vi "save digital settings.vi"(8 "error in (no error)":errorcluster, 11 "Digital Signal":T1={"DAQ Board Name"="DAQ_Simu1", "Port Digitales"=[], "rate"=1000.0, "Tiempo"=100}) -> (0 "error out":errorcluster)   [LabVIEW 2020, in "Settings.lvlib"]
uses:
  Settings.lvlib
  Digital typeSignal--cluster.ctl
  <vilib>/drjdpowell/SQLite Library/SQL Connection/Open (path).vi
  <vilib>/drjdpowell/SQLite Library/SQL Connection/Open (string).vi
  <vilib>/AdvancedString/Path To Command Line String.vi
  <vilib>/drjdpowell/SQLite Library/SQL Connection/Execute SQL (1D String).vi
  <vilib>/drjdpowell/SQLite Library/SQL Connection/Connection.lvclass
  <vilib>/drjdpowell/SQLite Library/SQLite.lvlib
panel:
  out "delimited string":string
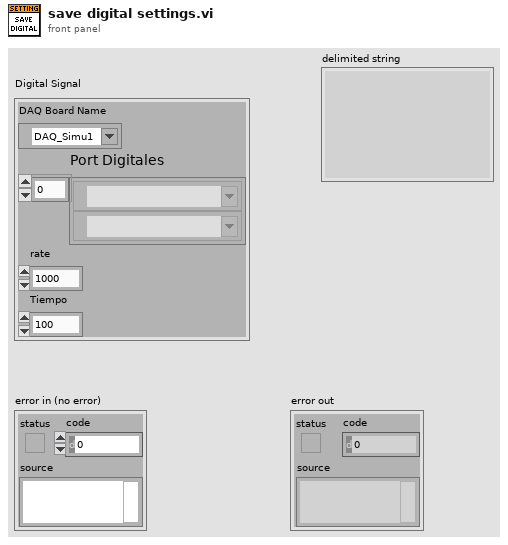
[diagram p1: front panel]
types:
  T1 = typedef "Digital typeSignal--cluster.ctl" = cluster{"DAQ Board Name":tag, "Port Digitales":tag[], "rate":dbl, "Tiempo":i32}
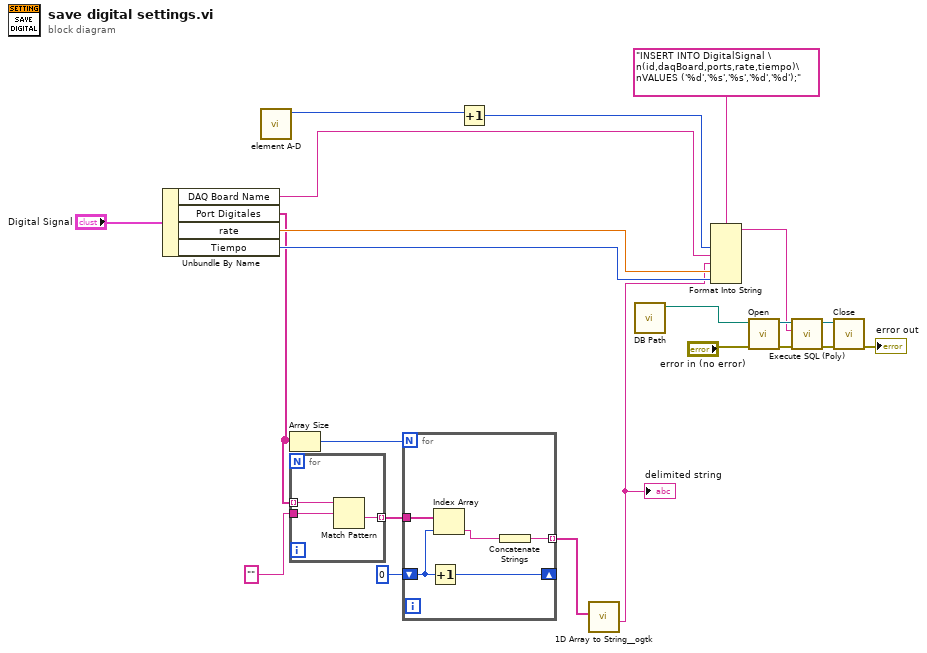
[diagram p0: block diagram]
diagram:
  n1 = Unbundle By Name("Digital Signal") -> ("DAQ Board Name"=w15:tag, "Port Digitales"=w2:tag[], "rate"=w12:dbl, "Tiempo"=w11:i32)
  n2 = call "element A-D.vi"() -> ("max(x,y)"=w8:i64)  [unwired: 10 in, 1 out]
  n3 = Array Size(array=w2) -> (size(s)=w6:i32)
  n4 = for {
    tunnel: [w25] -> w5 mode=indexing
    tunnel: "" ("regular expression") -> [w24]
    tunnel: w2 -> [w23] mode=indexing
    n5 = Match Pattern(string=w23, regular expression=w24) -> (after substring=w25:string)  [unwired: 1 in, 3 out]
  }
  n6 = for {
    N: w6 -> [_]
    shift-right: [w28] -> _
    shift-left: 0 -> [w29]
    tunnel: w5 -> [w30]
    tunnel: [w26] -> w7 mode=indexing
    n7 = Increment(x=w29) -> (x+1=w28:i32)
    n8 = Index Array(array=w30, index=w29) -> (element=w27:string)
    n9 = Concatenate Strings(w27) -> (w26:string)
  }
  n10 = Increment(x=w8) -> (x+1=w13:i64)
  n11 = call <userlib>:"1D Array to String__ogtk.vi"("Array of Strings"=w7) -> ("delimited string"=w1:string)  [unwired: 10 in]
  "delimited string" <- w1
  n12 = call "DB Path.vi"() -> ("DB path"=w14:path)  [unwired: 11 in]
  n13 = Format Into String(format string="INSERT INTO DigitalSignal \n(id,daqBoard,ports,rate,tiempo)\nVALUES ('%d','%s','%s','%d','%d');", w13, w15, w1, w12, w11) -> (resulting string=w9:string)  [unwired: 2 in, 1 out]
  n14 = call-poly <vilib>:"Open.vi"("error in (no error)"="error in (no error)", "db file"=w14) -> ("error out"=w22:errorcluster, "SQLite Connection"=w21:refnum<class "Connection.lvclass">)  [unwired: 8 in]
  n15 = call-poly <vilib>:"Execute SQL (Poly).vi"("error in (no error)"=w22, "SQL"=w9, "SQLite Connection in"=w21) -> ("error out"=w19:errorcluster, "SQLite Connection"=w20:refnum<class "Connection.lvclass">)  [unwired: 5 in, 2 out]
  n16 = call-dynamic "Close.vi"("error in (no error)"=w19, "SQLite Connection in"=w20) -> ("error out"=→"error out":errorcluster)  [unwired: 9 in]
